vi "Write Numeric Range to Source (Base10 I8).vi"(4 "min":i8 format="%d bytes", 5 "<= max? (F)":bool, 6 "max":i8 format="%d bytes", 7 ">= min? (F)":bool, 9 "offset":i32, 10 "value":i8 format="%d bytes", 11 "error in":errorcluster) -> (1 "new offset":i32, 3 "error out":errorcluster)   [LabVIEW 2017, in "Static Error Handling.lvlib"]
doc: "Writes a string in the form of <b>min</b> <=/< <b>value</b> <=/< <b>max</b> to the source string of the provided <b>error cluster</b> at the specified <b>offset</b>."
uses:
  Static Error Handling.lvlib
  Write Numeric Scalar to Source (Base10 I8).vi
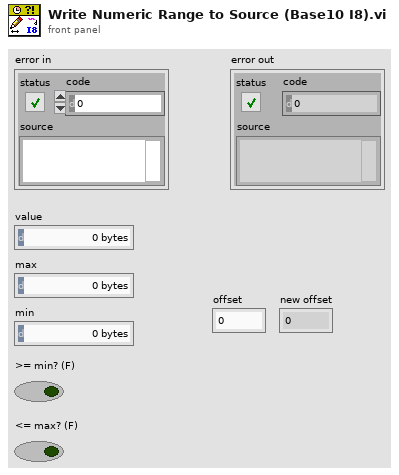
[diagram p1: front panel]
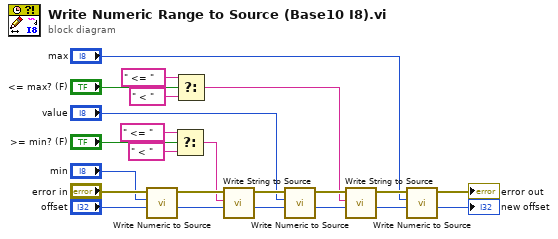
[diagram p0: block diagram]
diagram:
  n1 = call-poly "Write Numeric to Source.vi"("offset"="offset", "value"="min", "error in"="error in") -> ("new offset"=w22:i32, "error out"=w23:errorcluster)  [unwired: 7 in]
  n2 = Select(t=" <= ", s=">= min? (F)", f=" < ") -> (s? t:f=w7:string)
  n3 = Select(t=" <= ", s="<= max? (F)", f=" < ") -> (s? t:f=w1:string)
  n4 = call "Write String to Source.vi"("offset"=w22, "string"=w7, "error in"=w23) -> ("new offset"=w20:i32, "error out"=w21:errorcluster)  [unwired: 7 in]
  n5 = call-poly "Write Numeric to Source.vi"("offset"=w20, "value"="value", "error in"=w21) -> ("new offset"=w18:i32, "error out"=w19:errorcluster)  [unwired: 7 in]
  n6 = call "Write String to Source.vi"("offset"=w18, "string"=w1, "error in"=w19) -> ("new offset"=w16:i32, "error out"=w17:errorcluster)  [unwired: 7 in]
  n7 = call-poly "Write Numeric to Source.vi"("offset"=w16, "value"="max", "error in"=w17) -> ("new offset"=→"new offset":i32, "error out"=→"error out":errorcluster)  [unwired: 7 in]
